vi "myxmlparser-minimum working sample.vi"() -> ()   [LabVIEW 2011]
doc: "This example demonstrates how to query an XML document by using an XPath expression and returns all the nodes that match the XPath expression."
uses:
  <vilib>/xml/Close Reference(Node).vi
  Program Files (x86)/National Instruments/LabVIEW 2011/resource/objmgr/DOMUserDefRef.rc
  <vilib>/xml/NI_XML.lvlib
panel:
  out "value":cluster{dbl, dbl, dbl, dbl, bool, dbl, dbl}={10.0, -10.0, 22.4, 0.0, TRUE, 60.0, 10.0}
  out "xml string":string="<Cluster>\r\n<Name></Name>\r\n<NumElts>7</NumElts>\r\n<DBL>\r\n<Name></Name>\r\n<Val>0.00000000000000</Val>\r\n</DBL>\r\n<DBL>\r\n<Name></Name>\r\n<Val>0.00000000000000</Val>\r\n</DBL>\r\n<DBL>\r\n<Name></Name>\r\n<Val>0.00000000000000</Val>\r\n</DBL>\r\n<DBL>\r\n<Name></Name>\r\n<Val>0.00000000000000</Val>\r\n</DBL>\r\n<Boolean>\r\n<Name></Name>\r\n<Val>1</Val>\r\n</Boolean>\r\n<DBL>\r\n<Name></Name>\r\n<Val>0.00000000000000</Val>\r\n</DBL>\r\n<DBL>\r\n<Name></Name>\r\n<Val>0.00000000000000</Val>\r\n</DBL>\r\n</Cluster>\r\n"
  out "element":string="<Cluster>\n        <Name/>\n        <NumElts>7</NumElts>\n        <DBL>\n          <Name>max</Name>\n          <Val>10</Val>\n        </DBL>\n        <DBL>\n          <Name>min</Name>\n          <Val>-10</Val>\n        </DBL>\n        <DBL>\n          <Name>factor_a</Name>\n          <Val>22.4</Val>\n        </DBL>\n        <DBL>\n          <Name>factor_b</Name>\n          <Val>0.0</Val>\n        </DBL>\n        <Boolean>\n          <Name>lowpass</Name>\n          <Val>1</Val>\n        </Boolean>\n        <DBL>\n          <Name>lowpassfreq</Name>\n          <Val>60</Val>\n        </DBL>\n        <DBL>\n          <Name>excitation</Name>\n          <Val>10</Val>\n        </DBL>\n      </Cluster>"
  in  "index":i32
  in  "XPath expression":string="/SC0/mod0/ai0/Cluster"
  in  "XML document":string="<?xml version=\"1.0\" ?>\n<SC0>\n  <mod0>\n    <ai1>\n      <Cluster>\n        <Name></Name>\n        <NumElts>7</NumElts>\n        <DBL>\n          <Name>max</Name>\n          <Val>10</Val>\n        </DBL>\n        <DBL>\n          <Name>min</Name>\n          <Val>-10</Val>\n        </DBL>\n        <DBL>\n          <Name>factor_a</Name>\n          <Val>22.4</Val>\n        </DBL>\n        <DBL>\n          <Name>factor_b</Name>\n          <Val>0.0</Val>\n        </DBL>\n        <Boolean>\n          <Name>lowpass</Name>\n          <Val>1</Val>\n        </Boolean>\n        <DBL>\n          <Name>lowpassfreq</Name>\n          <Val>60</Val>\n        </DBL>\n        <DBL>\n          <Name>excitation</Name>\n          <Val>0.4</Val>\n        </DBL>\n      </Cluster>\n      <type>VoltageInputExtExc</type>\n      <name>234</name>\n    </ai1>\n    <ai0>\n      <Cluster>\n        <Name></Name>\n        <NumElts>7</NumElts>\n        <DBL>\n          <Name>max</Name>\n          <Val>10</Val>\n        </DBL>\n        <DBL>\n          <Name>min</Name>\n          <Val>-10</Val>\n        </DBL>\n        <DBL>\n          <Name>factor_a</Name>\n          <Val>22.4</Val>\n        </DBL>\n        <DBL>\n          <Name>factor_b</Name>\n          <Val>0.0</Val>\n        </DBL>\n        <Boolean>\n          <Name>lowpass</Name>\n          <Val>1</Val>\n        </Boolean>\n        <DBL>\n          <Name>lowpassfreq</Name>\n          <Val>60</Val>\n        </DBL>\n        <DBL>\n          <Name>excitation</Name>\n          <Val>10</Val>\n        </DBL>\n      </Cluster>\n      <type>VoltageInputIntExc</type>\n      <name>234</name>\n    </ai0>\n  </mod0>\n</SC0>\n"
  out "Result Array":string[](array[string])=["<Cluster>\n        <Name/>\n        <NumElts>7</NumElts>\n        <DBL>\n          <Name>max</Name>\n          <Val>10</Val>\n        </DBL>\n        <DBL>\n          <Name>min</Name>\n          <Val>-10</Val>\n        </DBL>\n        <DBL>\n          <Name>factor_a</Name>\n          <Val>22.4</Val>\n        </DBL>\n        <DBL>\n          <Name>factor_b</Name>\n          <Val>0.0</Val>\n        </DBL>\n        <Boolean>\n          <Name>lowpass</Name>\n          <Val>1</Val>\n        </Boolean>\n        <DBL>\n          <Name>lowpassfreq</Name>\n          <Val>60</Val>\n        </DBL>\n        <DBL>\n          <Name>excitation</Name>\n          <Val>10</Val>\n        </DBL>\n      </Cluster>"]
  # "This example demonstrates how to query an XML document by using an XPath expression and returns all the nodes that \nmatch the XPath expression."
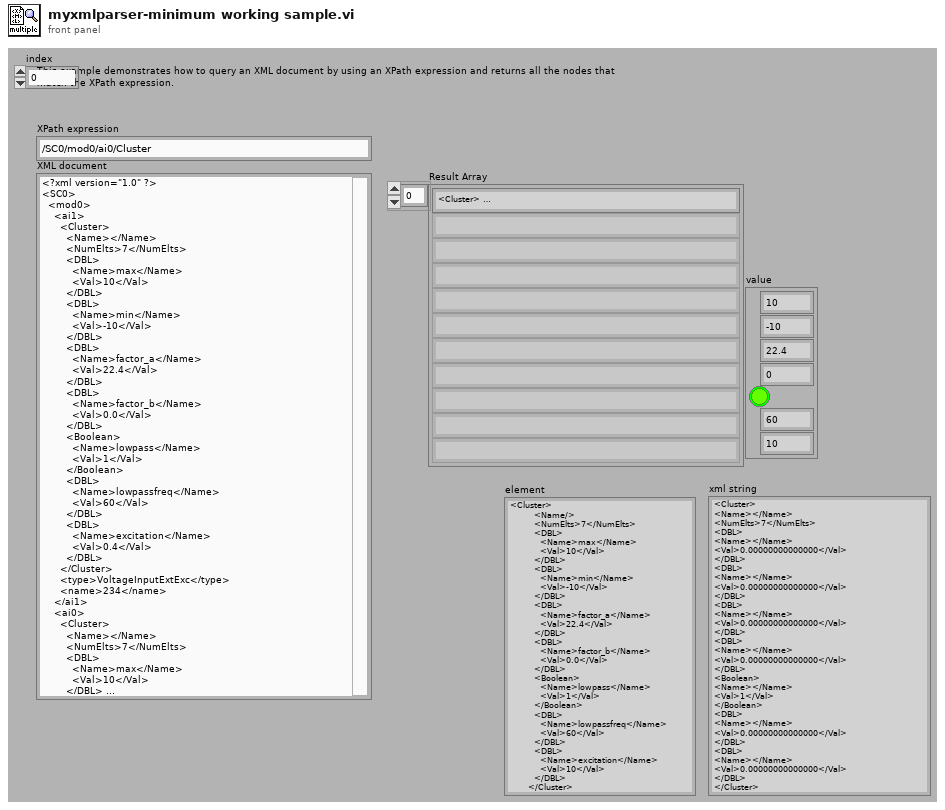
[diagram p1: front panel]
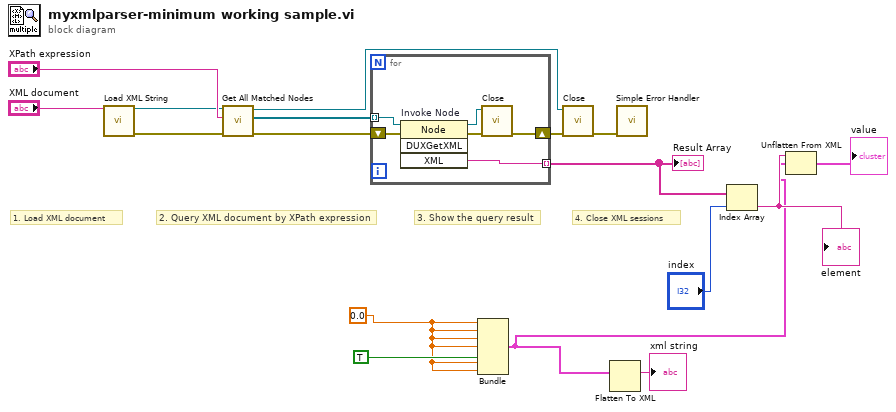
[diagram p0: block diagram]
diagram:
  w5 = 0.0
  # "4. Close XML sessions"
  # "3. Show the query result"
  # "2. Query XML document by XPath expression"
  # "1. Load XML document"
  n1 = call <vilib>:"Load XML String.vi"("XML string"="XML document") -> ("DOM document out"=w12:refnum<k20>, "error out"=w14:errorcluster)  [unwired: 1 in, 12 out]
  n2 = call <vilib>:"Get All Matched Nodes.vi"("error in (no error)"=w14, "XPath expression"="XPath expression", "node in"=w12) -> ("error out"=w15:errorcluster, "node result array"=w16:refnum<k20>[], "node out"=w10:refnum<k20>)  [unwired: 6 out]
  n3 = for {
    tunnel: w16 -> [w19] mode=indexing
    shift-right: [w21] -> w11
    shift-left: w15 -> [w20]
    tunnel: [w18] -> w8 mode=indexing
    n4 = invoke on="Invoke Node" class="Node" method="DUXGetXML"(reference=w19, error in=w20) -> (reference out=w22:refnum<k20>, error out=w23:errorcluster, "XML"=w18:string)  [unwired: 2 in, 1 out]
    n5 = call-poly <vilib>:"Close.vi"("error in (no error)"=w23, "node"=w22) -> ("error out"=w21:errorcluster)  [unwired: 7 out]
  }
  "Result Array" <- w8
  n6 = Bundle(w5, w5, w5, w5, TRUE, w5, w5) -> (w2:cluster{dbl, dbl, dbl, dbl, bool, dbl, dbl})  [unwired: 1 in]
  n7 = call-poly <vilib>:"Close.vi"("error in (no error)"=w11, "node"=w10) -> ("error out"=w9:errorcluster)  [unwired: 7 out]
  n8 = Flatten To XML(anything=w2) -> (xml string=→"xml string":string)
  n9 = call <vilib>:"Simple Error Handler.vi"("error in (no error)"=w9) -> ()  [unwired: 1 in, 8 out]
  n10 = Index Array(array=w8, index="index") -> (element=w4:string)
  "element" <- w4
  n11 = Unflatten From XML(xml string=w4, type=w2) -> (value=→"value":cluster{dbl, dbl, dbl, dbl, bool, dbl, dbl})  [unwired: 1 in, 1 out]
